vi "Convert to Searchable Web Address.vi"(8 "error in":errorcluster, 11 "Data":T1) -> (0 "error out":errorcluster, 3 "Data Out":T1)   [LabVIEW 2014]
uses:
  Controls/Data.ctl
  Controls/FP Control Refs.ctl
  Controls/Property.ctl
  Controls/Address.ctl
  Controls/Filter Criteria.ctl
  Controls/Fields.ctl
  Controls/Operator.ctl
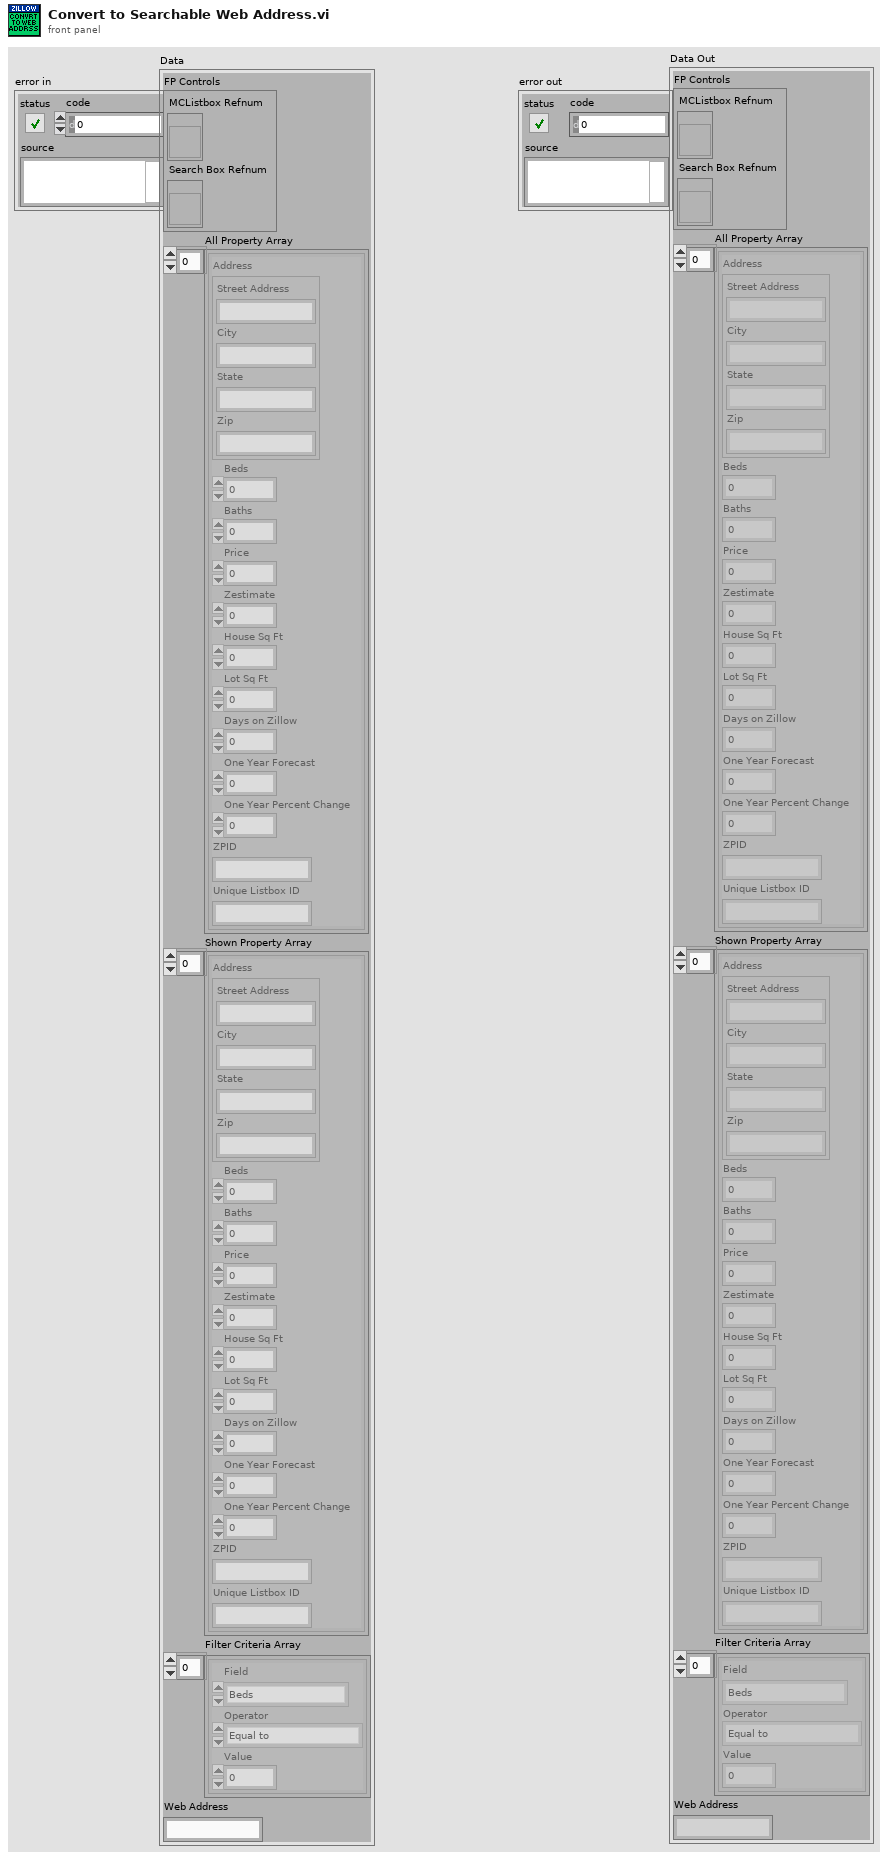
[diagram p1: front panel]
types:
  T1 = typedef "Data.ctl" = cluster{"FP Controls":T2, "All Property Array":T3[], "Shown Property Array":T3[], "Filter Criteria Array":T5[], "Web Address":string}
  T2 = typedef "FP Control Refs.ctl" = cluster{"MCListbox Refnum":refnum<vi>, "Search Box Refnum":refnum<vi>}
  T3 = typedef "Property.ctl" = cluster{"Address":T4, "Beds":dbl, "Baths":dbl, "Price":dbl, "Zestimate":dbl, "House Sq Ft":dbl, "Lot Sq Ft":dbl, "Days on Zillow":dbl, "One Year Forecast":dbl, "One Year Percent Change":dbl, "ZPID":string, "Unique Listbox ID":string}
  T4 = typedef "Address.ctl" = cluster{"Street Address":string, "City":string, "State":string, "Zip":string}
  T5 = typedef "Filter Criteria.ctl" = cluster{"Field":T6, "Operator":T7, "Value":dbl}
  T6 = typedef "Fields.ctl" = enum16{"Beds", "Baths", "Price", "Zestimate", "House Sq Ft", "Lot Sq Ft", "Days on Zillow", "One Year Forecast", "One Year Percent Change"}
  T7 = typedef "Operator.ctl" = enum16{"Equal to", "Greater than (or equal)", "Less than (or equal)", "Not Equal to"}
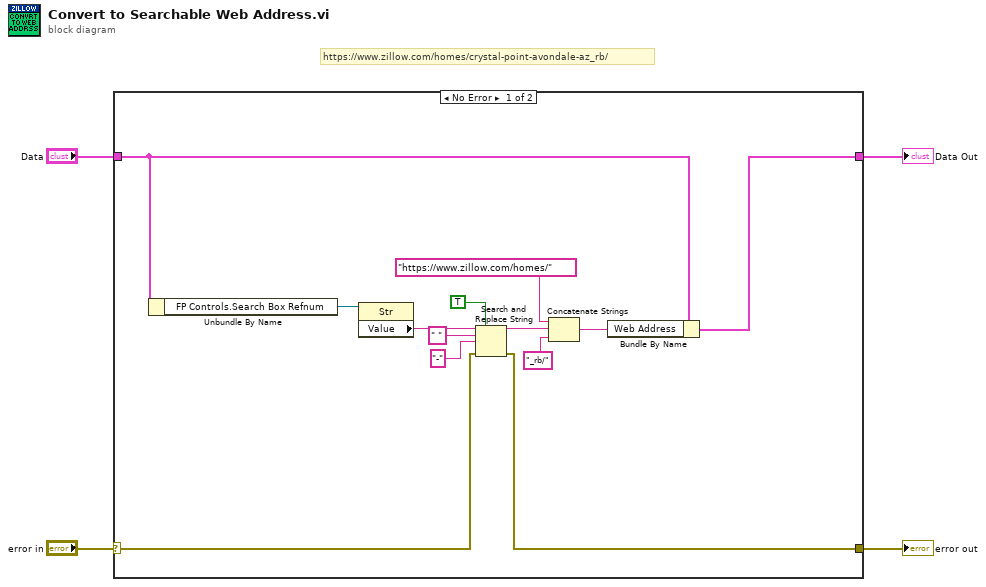
[diagram p0: block diagram]
diagram:
  # "https://www.zillow.com/homes/crystal-point-avondale-az_rb/"
  n1 = case shown="No Error" "error in" {
    selector: "error in" -> [w6 w19]
    tunnel: [w5 w19] -> w3
    tunnel: "Data" -> [w17 w18]
    tunnel: [w16 w18] -> w1
    frame No Error {
      n2 = Unbundle By Name(w17) -> ("FP Controls.Search Box Refnum"=w15:refnum<vi>)
      n3 = property class="Str"(reference=w15) -> ("Value"=w13:string)  [unwired: 1 in, 2 out]
      n4 = Search and Replace String(replace all?=TRUE ("replace all? (F)"), input string=w13, search string=" ", replace string="-" ("replace string (\"\")"), error in=w6) -> (result string=w10:string, error out=w5:errorcluster)  [unwired: 3 in, 2 out]
      n5 = Concatenate Strings("https://www.zillow.com/homes/", w10, "_rb/" ("replace string (\"\")")) -> (w8:string)
      n6 = Bundle By Name(cluster=w17, "Web Address"=w8) -> (w16:T1)
    }
    frame Error {
    }
  }
  "error out" <- w3
  "Data Out" <- w1
